vi "Read Sub Panel Mesj.vi"(8 "error in (no error)":errorcluster, 11 "Mensajes Actor in":refnum<class "Mensajes Actor.lvclass">) -> (0 "error out":errorcluster, 2 "Sub Panel Mesj":refnum<vi>, 3 "Mensajes Actor out":refnum<class "Mensajes Actor.lvclass">)   [LabVIEW 2019, in "Mensajes Actor.lvlib" / "Mensajes Actor.lvclass"]
uses:
  Mensajes Actor.lvclass
  Mensajes Actor.lvclass/Mensajes Actor.ctl
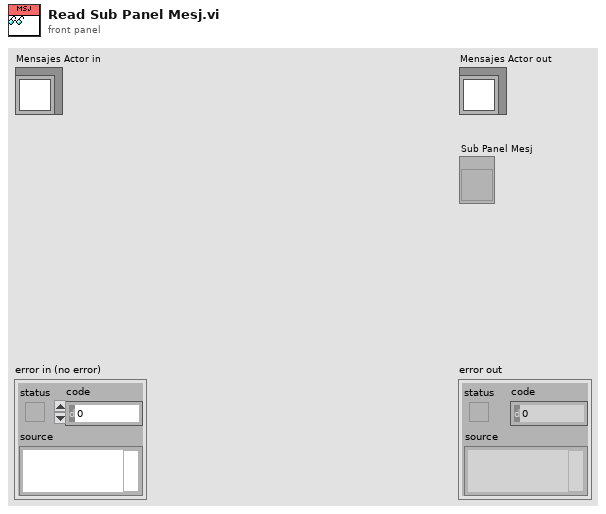
[diagram p1: front panel]
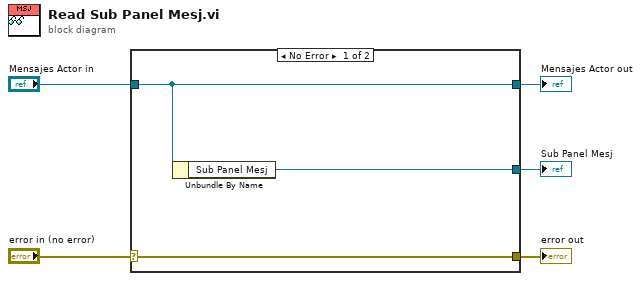
[diagram p0: block diagram]
diagram:
  n1 = case shown="No Error" "error in (no error)" {
    selector: "error in (no error)" -> [w8 w9]
    tunnel: [w8 w9] -> w4
    tunnel: [w7 w10] -> w2
    tunnel: "Mensajes Actor in" -> [w7 w10]
    tunnel: [w6 _] -> w1
    frame No Error {
      n2 = Unbundle By Name(w7) -> ("Sub Panel Mesj"=w6:refnum<vi>)
    }
    frame Error {
    }
  }
  "error out" <- w4
  "Mensajes Actor out" <- w2
  "Sub Panel Mesj" <- w1
